vi "Check.vi"() -> ()   [LabVIEW 2019]
uses:
  Z_source.ctl
  Heating/ctl/Z_Hswitch_little/Y_SourceInd.ctl
  Z_HSw.lvclass
  Z_HSw.lvclass/Z_HSw.ctl
  Heating/ctl/Z_Hswitch_little/Z_Hswitch_little.xctl
panel:
  out "Z1 ind":T1
  in  "Z_Source":T2
  in  "connect":bool
  in  "stop":bool
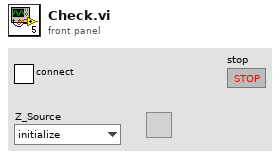
[diagram p1: front panel]
types:
  T1 = typedef "Heating.lvlib/Z_Hswitch_little.xctl/Y_SourceInd.ctl" = u8
  T2 = typedef "Z_source.ctl" = enum8{"initialize", "local disabled", "local hand", "hand", "auto", "dist"}
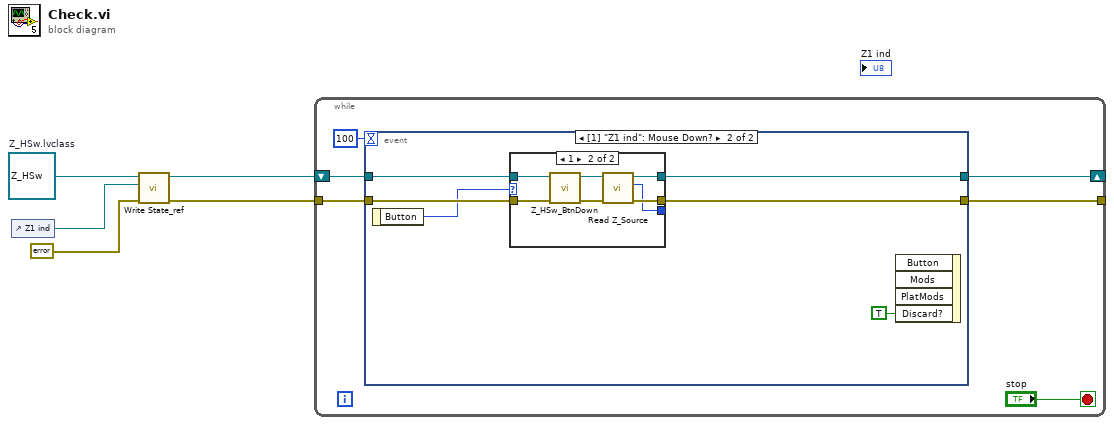
[diagram p0: block diagram]
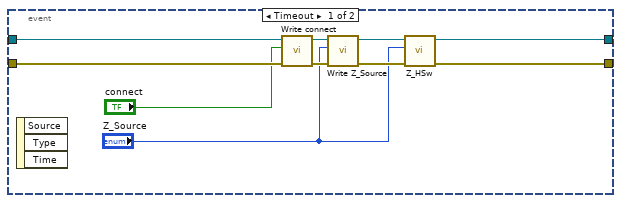
[diagram p2: hidden frame]
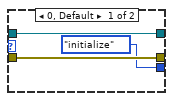
[diagram p3: hidden frame]
diagram:
  w5 = refnum<class "Z_HSw.lvclass"> refnum  # Z_HSw.lvclass
  n1 = control-ref of="Z1 ind"() -> (w1:refnum<vi>)
  n2 = call "Write State_ref.vi"("error in (no error)"=errorcluster {"status"=FALSE, "code"=0, "source"=""}, "State_ref"=w1, "Z_HSw in"=w5) -> ("error out"=w3:errorcluster, "Z_HSw out"=w4:refnum<class "Z_HSw.lvclass">)  [unwired: 7 in]
  n3 = while {
    tunnel: w3 -> [w7]
    shift-right: [w11] -> _
    shift-left: w4 -> [w9]
    tunnel: [w6] -> _
    stop <- "stop" stop-if-true
    n4 = event shown="[1] \"Z1 ind\": Mouse Down?" {
      selector: _ -> [_ _]
      dyn-events: _ -> [_ _]
      timeout: 100 -> [_ _]
      tunnel: [w20 w23] -> w11
      tunnel: w9 -> [w19 w26]
      tunnel: w7 -> [w16 w25]
      tunnel: [w21 w22] -> w6
      event Timeout {
        n5 = event-data() -> ()  [unwired: 1 in, 3 out]
        n6 = call "Write connect.vi"("error in (no error)"=w16, "connect"="connect", "Z_HSw in"=w19) -> ("error out"=w15:errorcluster, "Z_HSw out"=w17:refnum<class "Z_HSw.lvclass">)  [unwired: 7 in]
        n7 = call "Write Z_Source.vi"("error in (no error)"=w15, "Z_Source"="Z_Source", "Z_HSw in"=w17) -> ("error out"=w14:errorcluster, "Z_HSw out"=w18:refnum<class "Z_HSw.lvclass">)  [unwired: 7 in]
        n8 = call "Z_HSw.vi"("error in (no error)"=w14, "Z_Source"="Z_Source", "Z_HSw_in"=w18) -> ("error out"=w21:errorcluster, "Z_HSw_out"=w20:refnum<class "Z_HSw.lvclass">)  [unwired: 7 in]
      }
      event Mouse Down? {
        n9 = event-data() -> ("Button"=w24:u16)  [unwired: 1 in]
        n10 = case shown="1" w24 {
          tunnel: [w30 w31] -> w23
          tunnel: w26 -> [w30 w32]
          tunnel: w25 -> [w29 w37]
          tunnel: [w29 w36] -> w22
          tunnel: [Z_source."initialize" ("Z_Source") w35] -> _
          frame 0, Default {
          }
          frame 1 {
            n11 = call "Z_HSw_BtnDown.vi"("error in (no error)"=w37, "Z_HSw_in"=w32) -> ("error out"=w33:errorcluster, "Z_HSw_out"=w34:refnum<class "Z_HSw.lvclass">)  [unwired: 7 in, 1 out]
            n12 = call "Read Z_Source.vi"("error in (no error)"=w33, "Z_HSw in"=w34) -> ("error out"=w36:errorcluster, "Z_Source"=w35:T2, "Z_HSw out"=w31:refnum<class "Z_HSw.lvclass">)  [unwired: 7 in]
          }
        }
        n13 = event-data("Discard?"=TRUE) -> ()  [unwired: 4 in, 1 out]
      }
    }
  }
